vi "test17-LosslessRegisterStateMultipleTimes.vi"(8 "error in (no error)":errorcluster, 11 "TestCase in":refnum<class "testcase-CSMBroadcast.lvclass">) -> (0 "error out":errorcluster, 3 "TestCase out":refnum<class "testcase-CSMBroadcast.lvclass">)   [LabVIEW 2017, in "testcase-CSMBroadcast.lvclass"]
uses:
  testcase-CSMBroadcast.lvclass
  bc269a46-fbd8-4fbd-ac76-06990d02385a.vi
  8d37a2f4-20d8-4102-818c-5a8acec6f80e.vi
  src/user.lib/_NEVSTOP/Communicable State Machine(CSM)/AdvanceAPI/CSM - Get Module Attribute.vi
  <vilib>/addons/_JKI Toolkits/VI Tester/TestCase.llb/TestCase.lvclass
  src/user.lib/_NEVSTOP/Communicable State Machine(CSM)/Communicable State Machine.lvlib
  C:/Program Files (x86)/National Instruments/LabVIEW 2017/vi.lib/addons/_JKI Toolkits/VI Tester/TestCase.llb/TestCase.lvclass
panel:
  out "LoopCount":i32
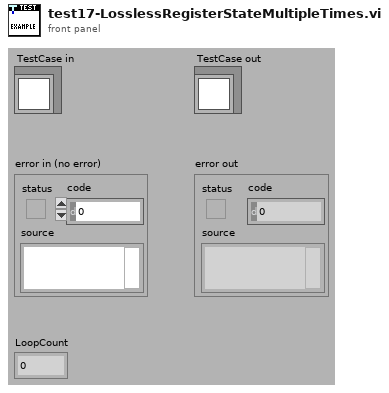
[diagram p1: front panel]
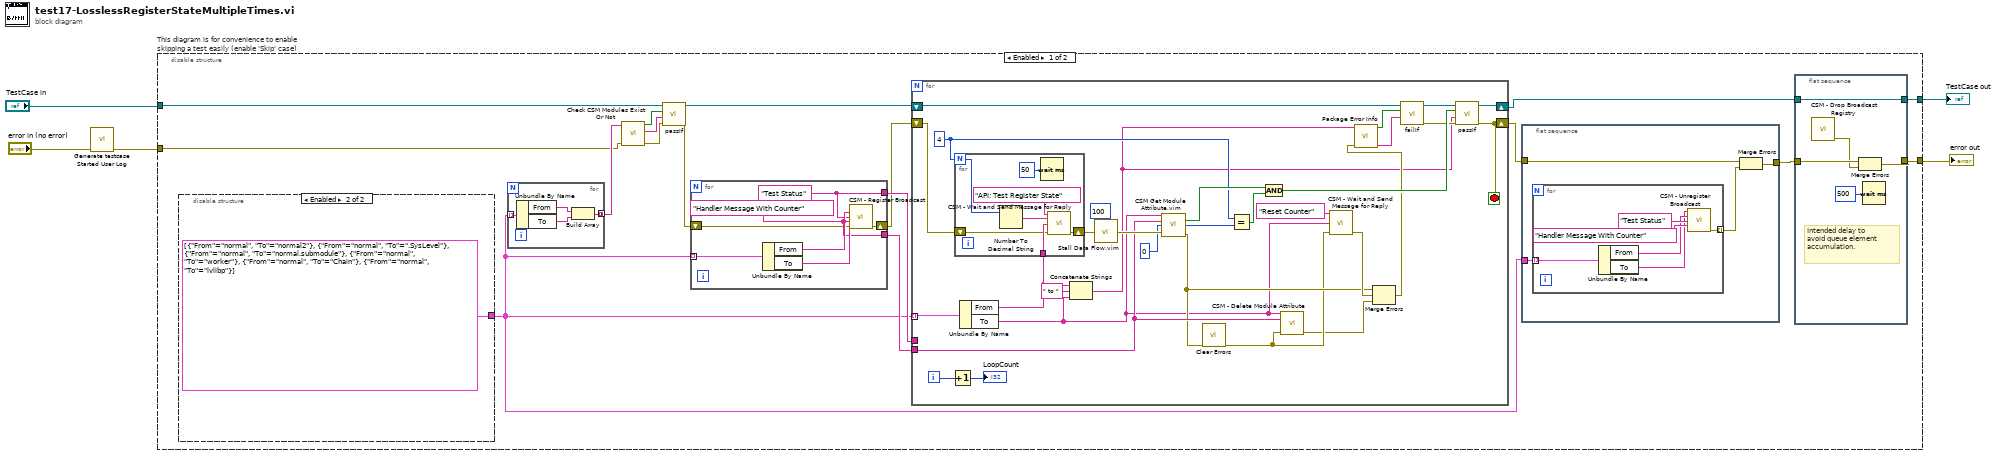
[diagram p0: block diagram]
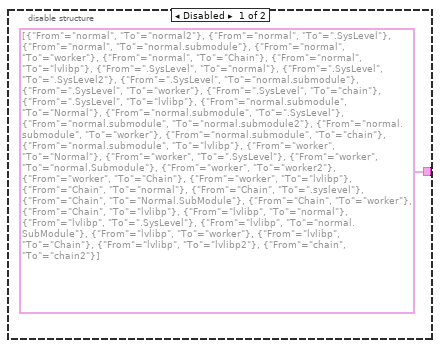
[diagram p2: hidden frame]
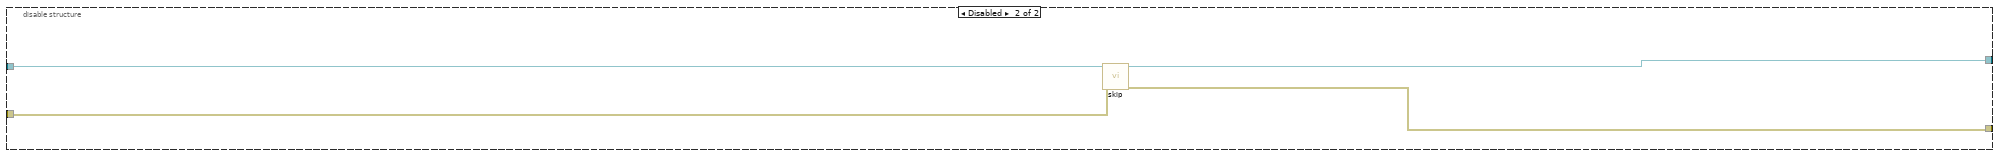
[diagram p3: hidden frame]
diagram:
  n1 = call "Generate testcase Started User Log.vi"("Error In"="error in (no error)") -> ("error out"=w1:errorcluster)  [unwired: 10 in]
  n2 = disable-structure "This diagram is for convenience to enable skipping a test easily (enable 'Skip' case)" shown="Enabled" {
    disable-tunnel: "TestCase in" -> [w11 w92]
    disable-tunnel: [w17 w90] -> w3
    disable-tunnel: [w20 w91] -> w2
    disable-tunnel: w1 -> [w9 w89]
    frame Enabled {
      n3 = disable-structure shown="Enabled" {
        disable-tunnel: [cluster{"From":string, "To":string}[] [{"From"="normal", "To"="normal2"}, {"From"="normal", "To"=".SysLevel"}, {"From"="normal", "To"="normal.submodule"}, {"From"="normal", "To"="worker"}, {"From"="normal", "To"="Chain"}, {"From"="normal", "To"="lvlibp"}, {"From"=".SysLevel", "To"="normal"}, {"From"=".SysLevel", "To"=".SysLevel2"}, {"From"=".SysLevel", "To"="normal.submodule"}, {"From"=".SysLevel", "To"="worker"}, {"From"=".SysLevel", "To"="chain"}, {"From"=".SysLevel", "To"="lvlibp"}, {"From"="normal.submodule", "To"="Normal"}, {"From"="normal.submodule", "To"=".SysLevel"}, {"From"="normal.submodule", "To"="normal.submodule2"}, {"From"="normal.submodule", "To"="worker"}, {"From"="normal.submodule", "To"="chain"}, {"From"="normal.submodule", "To"="lvlibp"}, {"From"="worker", "To"="Normal"}, {"From"="worker", "To"=".SysLevel"}, {"From"="worker", "To"="normal.Submodule"}, {"From"="worker", "To"="worker2"}, {"From"="worker", "To"="Chain"}, {"From"="worker", "To"="lvlibp"}, {"From"="Chain", "To"="normal"}, {"From"="Chain", "To"=".syslevel"}, {"From"="Chain", "To"="Normal.SubModule"}, {"From"="Chain", "To"="worker"}, {"From"="Chain", "To"="lvlibp"}, {"From"="lvlibp", "To"="normal"}, {"From"="lvlibp", "To"=".SysLevel"}, {"From"="lvlibp", "To"="normal.SubModule"}, {"From"="lvlibp", "To"="worker"}, {"From"="lvlibp", "To"="Chain"}, {"From"="lvlibp", "To"="lvlibp2"}, {"From"="chain", "To"="chain2"}] cluster{"From":string, "To":string}[] [{"From"="normal", "To"="normal2"}, {"From"="normal", "To"=".SysLevel"}, {"From"="normal", "To"="normal.submodule"}, {"From"="normal", "To"="worker"}, {"From"="normal", "To"="Chain"}, {"From"="normal", "To"="lvlibp"}]] -> w6
        frame Disabled {
        }
        frame Enabled {
        }
      }
      n4 = for {
        tunnel: w6 -> [w28] mode=indexing
        tunnel: [w25] -> w14 mode=concatenating
        n5 = Unbundle By Name(w28) -> ("From"=w27:string, "To"=w26:string)
        n6 = Build Array(w27, w26) -> (w25:string[])
      }
      n7 = call "Check CSM Modules Exist Or Not.vi"("error in"=w9, "CSM names in"=w14) -> ("error out"=w12:errorcluster, "Debug string"=w13:string, "All Modules Exist?"=w15:bool)  [unwired: 7 in]
      n8 = call-dynamic "passIf.vi"("error in (no error)"=w12, "message (\"\")"=w13, "pass"=w15, "TestCase in"=w11) -> ("error out"=w8:errorcluster, "TestCase out"=w10:refnum<class "testcase-CSMBroadcast.lvclass">)  [unwired: 6 in]
      n9 = for {
        tunnel: w6 -> [w45] mode=indexing
        tunnel: [w41] -> w19
        tunnel: [w40] -> w16
        shift-right: [w42] -> w7
        shift-left: w8 -> [w39]
        w40 = "Handler Message With Counter" ("Response Message (If \"\", Same as Source Message)")
        w41 = "Test Status" ("Status")
        n10 = Unbundle By Name(w45) -> ("From"=w44:string, "To"=w43:string)
        n11 = call "CSM - Register Broadcast.vi"("CSM Name(Empty for Broadcast Event)"=w43, "Source CSM Name (* as Default)"=w44, "Trigger"=w41, "API (If \"\", Same as Trigger)"=w40, "Error In"=w39) -> ("error out"=w42:errorcluster)  [unwired: 9 in, 1 out]
      }
      n12 = for {
        tunnel: w6 -> [w81] mode=indexing
        shift-right: [w76] -> w18
        shift-left: w10 -> [w58]
        shift-right: [w74] -> w22
        shift-left: w7 -> [w61]
        tunnel: w19 -> [_]
        tunnel: w16 -> [w73]
        i -> [w72]
        stop <- w74 stop-if-true
        w68 = 4
        n13 = Increment(x=w72) -> (x+1=→"LoopCount":i32)
        n14 = Unbundle By Name(w81) -> ("From"=w54:string, "To"=w53:string)
        n15 = for {
          N: w68 -> [w83]
          tunnel: w54 -> [w86]
          shift-right: [w87] -> w80
          shift-left: w61 -> [w85]
          n16 = Number To Decimal String(number=w83) -> (decimal integer string=w84:string)  [unwired: 1 in]
          n17 = Wait (ms)(milliseconds to wait=u32 50) -> ()  [unwired: 1 out]
          n18 = call "CSM - Wait and Send Message for Reply.vi"("State"="API: Test Register State", "Arguments (\"\")"=w84, "Target Module"=w86, "Error In (No Error)"=w85) -> ("error out"=w87:errorcluster)  [unwired: 8 in, 3 out]
        }
        n19 = Concatenate Strings(w54, " to " ("string"), w53) -> (w51:string)
        n20 = call "Stall Data Flow.vim"("value in"=w80, "milliseconds to wait"=u32 100) -> ("value out"=w78:errorcluster)  [unwired: 1 out]
        n21 = call "CSM Get Module Attribute.vim"("CSM Name"=w53, "Attribute"=w73, "Default Value (Empty Variant)"=u32 0, "Error In"=w78) -> ("Found"=w77:bool, "Value"=w69:u32, "error out"=w64:errorcluster)  [unwired: 7 in, 2 out]
        n22 = call <vilib>:"Clear Errors.vi"("error in (no error)"=w64) -> ("error out"=w63:errorcluster)  [unwired: 5 in, 1 out]
        n23 = Equal?(x=w68, y=w69) -> (x = y?=w67:bool)
        n24 = Compound Arithmetic op=AND(w77, w67) -> (w75:bool)
        n25 = call "CSM - Delete Module Attribute.vi"("CSM Name"=w53, "Attribute"=w73, "Error In"=w63) -> ("error out"=w62:errorcluster)  [unwired: 9 in, 3 out]
        n26 = call "CSM - Wait and Send Message for Reply.vi"("State"="Reset Counter", "Target Module"=w53, "Error In (No Error)"=w63) -> ("error out"=w65:errorcluster)  [unwired: 9 in, 3 out]
        n27 = Merge Errors(w64, w65, w62) -> (w55:errorcluster)
        n28 = call "Package Error Info.vi"("error in"=w55, "String in"=w51) -> ("packed error info out"=w59:string, "error status"=w60:bool)  [unwired: 8 in]
        n29 = call-dynamic "failIf.vi"("message (\"\")"=w59, "fail"=w60, "TestCase in"=w58) -> ("error out"=w56:errorcluster, "TestCase out"=w57:refnum<class "testcase-CSMBroadcast.lvclass">)  [unwired: 7 in]
        n30 = call-dynamic "passIf.vi"("error in (no error)"=w56, "message (\"\")"=w51, "pass"=w75, "TestCase in"=w57) -> ("error out"=w74:errorcluster, "TestCase out"=w76:refnum<class "testcase-CSMBroadcast.lvclass">)  [unwired: 6 in]
      }
      n31 = flat-sequence {
        tunnel: w6 -> [w29]
        tunnel: w22 -> [w32]
        tunnel: [w31] -> w21
        frame #0 {
          n32 = for {
            tunnel: w29 -> [w33] mode=indexing
            tunnel: [w34] -> w30 mode=indexing
            n33 = Unbundle By Name(w33) -> ("From"=w36:string, "To"=w35:string)
            n34 = call "CSM - Unregister Broadcast.vi"("CSM Name(Empty for Broadcast Event)"=w35, "Source CSM Name (* as Default)"=w36, "Trigger"="Test Status" ("Status"), "API (\"*\" as Default)"="Handler Message With Counter" ("Response Message (If \"\", Same as Source Message)")) -> ("error out"=w34:errorcluster)  [unwired: 10 in, 1 out]
          }
          n35 = Merge Errors(w32, w30) -> (w31:errorcluster)
        }
      }
      n36 = flat-sequence {
        tunnel: w21 -> [w50]
        tunnel: [w49] -> w20
        tunnel: [w48] -> w17
        tunnel: w18 -> [w48]
        frame #0 {
          # "Intended delay to\navoid queue element\naccumulation."
          n37 = call "CSM - Drop Broadcast Registry.vi"() -> ("error out"=w47:errorcluster)  [unwired: 15 in]
          n38 = Merge Errors(w50, w47) -> (w49:errorcluster)
          n39 = Wait (ms)(milliseconds to wait=u32 500) -> ()  [unwired: 1 out]
        }
      }
    }
    frame Disabled {
      # "skip test result while test is under development"
      n40 = call <vilib>:"skip.vi"("error in (no error)"=w89, "TestCase in"=w92) -> ("error out"=w91:errorcluster, "TestCase out"=w90:refnum<class "testcase-CSMBroadcast.lvclass">)  [unwired: 8 in]
    }
  }
  "error out" <- w2
  "TestCase out" <- w3
